vi "Disabled.vi"(7 "Robot Mode":T2, 10 "Match Info":T1={"Autonomous Elapsed Seconds"=0.0, "TeleOp Elapsed Seconds"=0.0, "Disabled Elapsed Seconds"=0.0, "Visited Autonomous"=FALSE, "Visited TeleOp"=FALSE, "Visited Disabled"=FALSE, "Autonomous Settings"={"Autonomous Style"=enum."Independent", "VI Refnum"=refnum}}, 11 "Call Context":T3) -> ()   [LabVIEW 2011]
doc: "This VI is called each time a disabled packet is received from the DS. It is often used to prepare for the next robot mode, to calibrate sensors, etc."
uses:
  <vilib>/Rock Robotics/WPI/DriverStation/WPI_DriverStationDerivedRobotMode.ctl
  <vilib>/Rock Robotics/WPI/DriverStation/WPI_DriverStationRobotMode.ctl
  <vilib>/Rock Robotics/WPI/DriverStation/WPI_DriverStationMatch Info.ctl
  Robot Global Data.vi
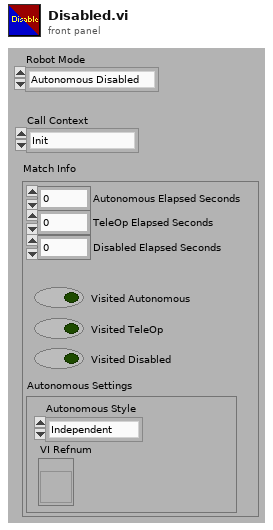
[diagram p1: front panel]
types:
  T1 = typedef "WPI_DriverStationMatch Info.ctl" = cluster{"Autonomous Elapsed Seconds":dbl, "TeleOp Elapsed Seconds":dbl, "Disabled Elapsed Seconds":dbl, "Visited Autonomous":bool, "Visited TeleOp":bool, "Visited Disabled":bool, "Autonomous Settings":cluster{"Autonomous Style":enum16{"Iterative", "Independent"}, "VI Refnum":refnum<vi>}}
  T2 = typedef "WPI_DriverStationRobotMode.ctl" = enum16{"Autonomous Disabled", "Autonomous Enabled", "Teleop Disabled", "Teleop Enabled", "Timeout", "Finish"}
  T3 = typedef "WPI_DriverStationDerivedRobotMode.ctl" = enum16{"Init", "Execute", "Stop"}
  T4 = typedef "WPI_EncoderDevRef.ctl" = cluster{"DevStatus":errorcluster, "EncoderIndex":T5, "CounterIndex":T6, "DistancePerCount":dbl, "Decoding Type":T7}
  T5 = typedef "FPGA_EncoderIdx.ctl" = enum8{"Enc 0", "Enc 1", "Enc 2", "Enc 3", "Invalid"}
  T6 = typedef "FPGA_CounterCtrSystemIndex.ctl" = enum8{"Ctr 0", "Ctr 1", "Ctr 2", "Ctr 3", "Ctr 4", "Ctr 5", "Ctr 6", "Ctr 7", "Invalid"}
  T7 = typedef "WPI_EncoderType.ctl" = enum16{"1x", "2x", "4x"}
  T8 = typedef "WPI_GyroDevRef.ctl" = cluster{"DevStatus":errorcluster, "Analog Module":T9, "Analog Channel":T10, "Offset":dbl, "Gain (VoltsPerDegree/Second)":dbl}
  T9 = typedef "FPGA_TypedefAnalogModule.ctl" = enum16{"Analog Module 1", "Analog Module 2"}
  T10 = typedef "FPGA_AIChannel.ctl" = enum8{"AI 1", "AI 2", "AI 3", "AI 4", "AI 5", "AI 6", "AI 7", "AI 8", "Invalid"}
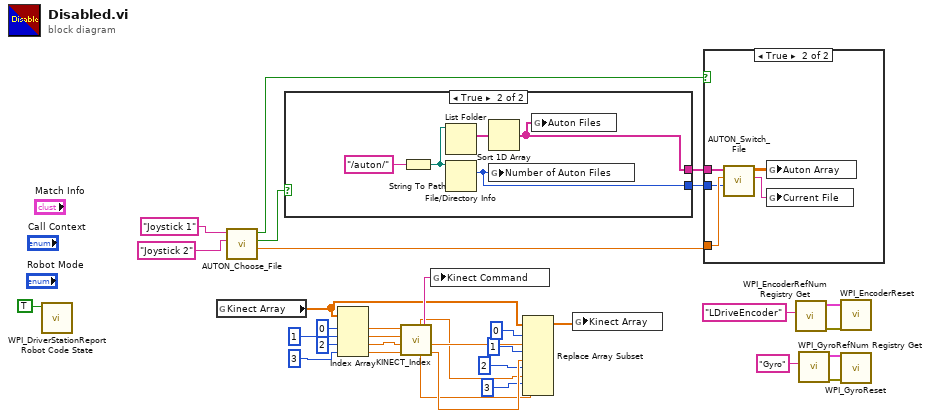
[diagram p0: block diagram]
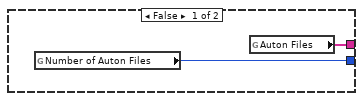
[diagram p3: hidden frame]
diagram:
  n1 = call <vilib>:"WPI_DriverStationReport Robot Code State.vi"("Disabled"=TRUE ("Autonomous")) -> ()  [unwired: 10 in, 1 out]
  n2 = global read "Robot Global Data.vi" "Kinect Array"() -> (w23:dbl[])
  n3 = call "AUTON_Choose_File.vi"("Joystick 2 Refnum"="Joystick 2" ("refnum name"), "Joystick 1 Refnum"="Joystick 1" ("refnum name")) -> ("Auton File"=w1:dbl, "Refresh"=w3:bool, "Allow Change"=w2:bool)  [unwired: 7 in]
  n4 = case shown="True" w3 {
    tunnel: [w34 w37] -> w12
    tunnel: [w35 w36] -> w13
    frame False {
      n5 = global read "Robot Global Data.vi" "Number of Auton Files"() -> (w34:i64)
      n6 = global read "Robot Global Data.vi" "Auton Files"() -> (w35:string[])
    }
    frame True {
      n7 = String To Path(string="/auton/") -> (path=w39:path)
      n8 = List Folder(path=w39) -> (filenames=w38:string[])  [unwired: 1 in, 5 out]
      n9 = File/Directory Info(path=w39) -> (size=w37:i64)  [unwired: 1 in, 6 out]
      n10 = Sort 1D Array(array=w38) -> (sorted array=w36:string[])
      n11 = global write "Robot Global Data.vi" "Number of Auton Files"(w37) -> ()
      n12 = global write "Robot Global Data.vi" "Auton Files"(w36) -> ()
    }
  }
  n13 = Index Array(array=w23, index #1=0 ("index"), index #2=1 ("index"), index #3=2 ("index"), index #4=3 ("index")) -> (element #1=w27:dbl, element #2=w26:dbl, element #3=w25:dbl, element #4=w24:dbl)
  n14 = call "KINECT_Index.vi"("Arm Drive Min in (Reverse)"=w24, "Arm Drive Max in (Forward)"=w25, "Z Wrist Left"=w26, "Z Wrist Right"=w27) -> ("Z Wrist Left"=w19:sgl, "Z Wrist Right"=w21:sgl, "Kinect Command"=w32:string, "Arm Drive Min out (Reverse)"=w15:dbl, "Arm Drive Max out (Forward)"=w16:dbl)  [unwired: 3 in]
  n15 = global write "Robot Global Data.vi" "Kinect Command"(w32) -> ()
  n16 = Replace Array Subset(array=w23, new element #1=w21, index #1=0 ("index"), new element #2=w19, index #2=1 ("index"), new element #3=w16, index #3=2 ("index"), new element #4=w15, index #4=3 ("index")) -> (w14:dbl[])
  n17 = global write "Robot Global Data.vi" "Kinect Array"(w14) -> ()
  n18 = case shown="True" w2 {
    tunnel: w1 -> [_ w43]
    tunnel: w13 -> [_ w42]
    tunnel: w12 -> [_ w41]
    frame False {
    }
    frame True {
      n19 = call "AUTON_Switch_File.vi"("Number of Auton Files"=w41, "Auton File"=w43, "Auton Files"=w42) -> ("Current File"=w44:string, "Auton Array"=w45:dbl[][])  [unwired: 7 in]
      n20 = global write "Robot Global Data.vi" "Auton Array"(w45) -> ()
      n21 = global write "Robot Global Data.vi" "Current File"(w44) -> ()
    }
  }
  n22 = call <vilib>:"WPI_EncoderRefNum Registry Get.vi"("refnum name"="LDriveEncoder") -> ("error out"=w11:errorcluster, "EncoderDevRef"=w10:T4)  [unwired: 9 in]
  n23 = call <vilib>:"WPI_GyroRefNum Registry Get.vi"("refnum name"="Gyro") -> ("error out"=w8:errorcluster, "GyroDevRef"=w9:T8)  [unwired: 9 in]
  n24 = call <vilib>:"WPI_EncoderReset.vi"("error in (no error)"=w11, "EncoderDevRef"=w10) -> ()  [unwired: 8 in, 2 out]
  n25 = call <vilib>:"WPI_GyroReset.vi"("error in (no error)"=w8, "GyroDevRef"=w9) -> ()  [unwired: 8 in, 2 out]
